vi "CREAT_SQL_TABLE.vi"() -> ()   [LabVIEW 2017]
uses:
  <vilib>/addons/database/Auxilliary.llb/DB Tools DataTypes.ctl
  <vilib>/addons/database/Connection.llb/DB Tools Open Connec (Path).vi
  <vilib>/addons/database/NI_Database_API.lvlib
panel:
  out "columns":string[](array[string])
  out "column information":T2(array[cluster])
  out "error out":errorcluster
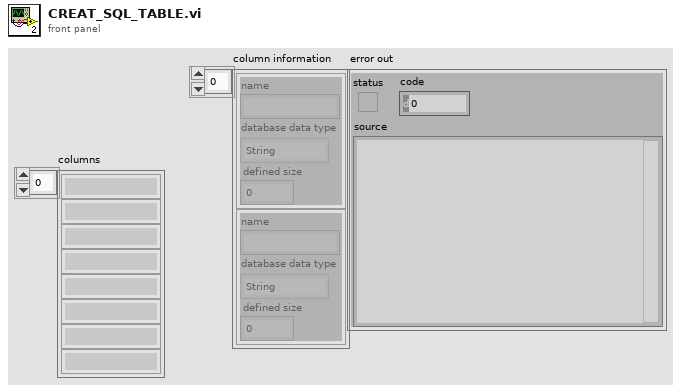
[diagram p1: front panel]
types:
  T1 = typedef "NI_Database_API.lvlib/DB Tools DataTypes.ctl" = enum16{"String", "Long (I32)", "Single (SGL)", "Double (DBL)", "Date/Time", "Binary"}
  T2 = cluster{"name":string, "database data type":T1, "defined size":i32}[]
  T3 = cluster{"name":string, "database data type":T1, "defined size":i32, "allow null?":bool}[]
  T4 = typedef "NI_Database_API.lvlib/Conn ObjectReference.ctl" = refnum<k1>
  T5 = cluster{"seconds since 1Jan1904":timestamp, "table":string, "table":string, "table":string}
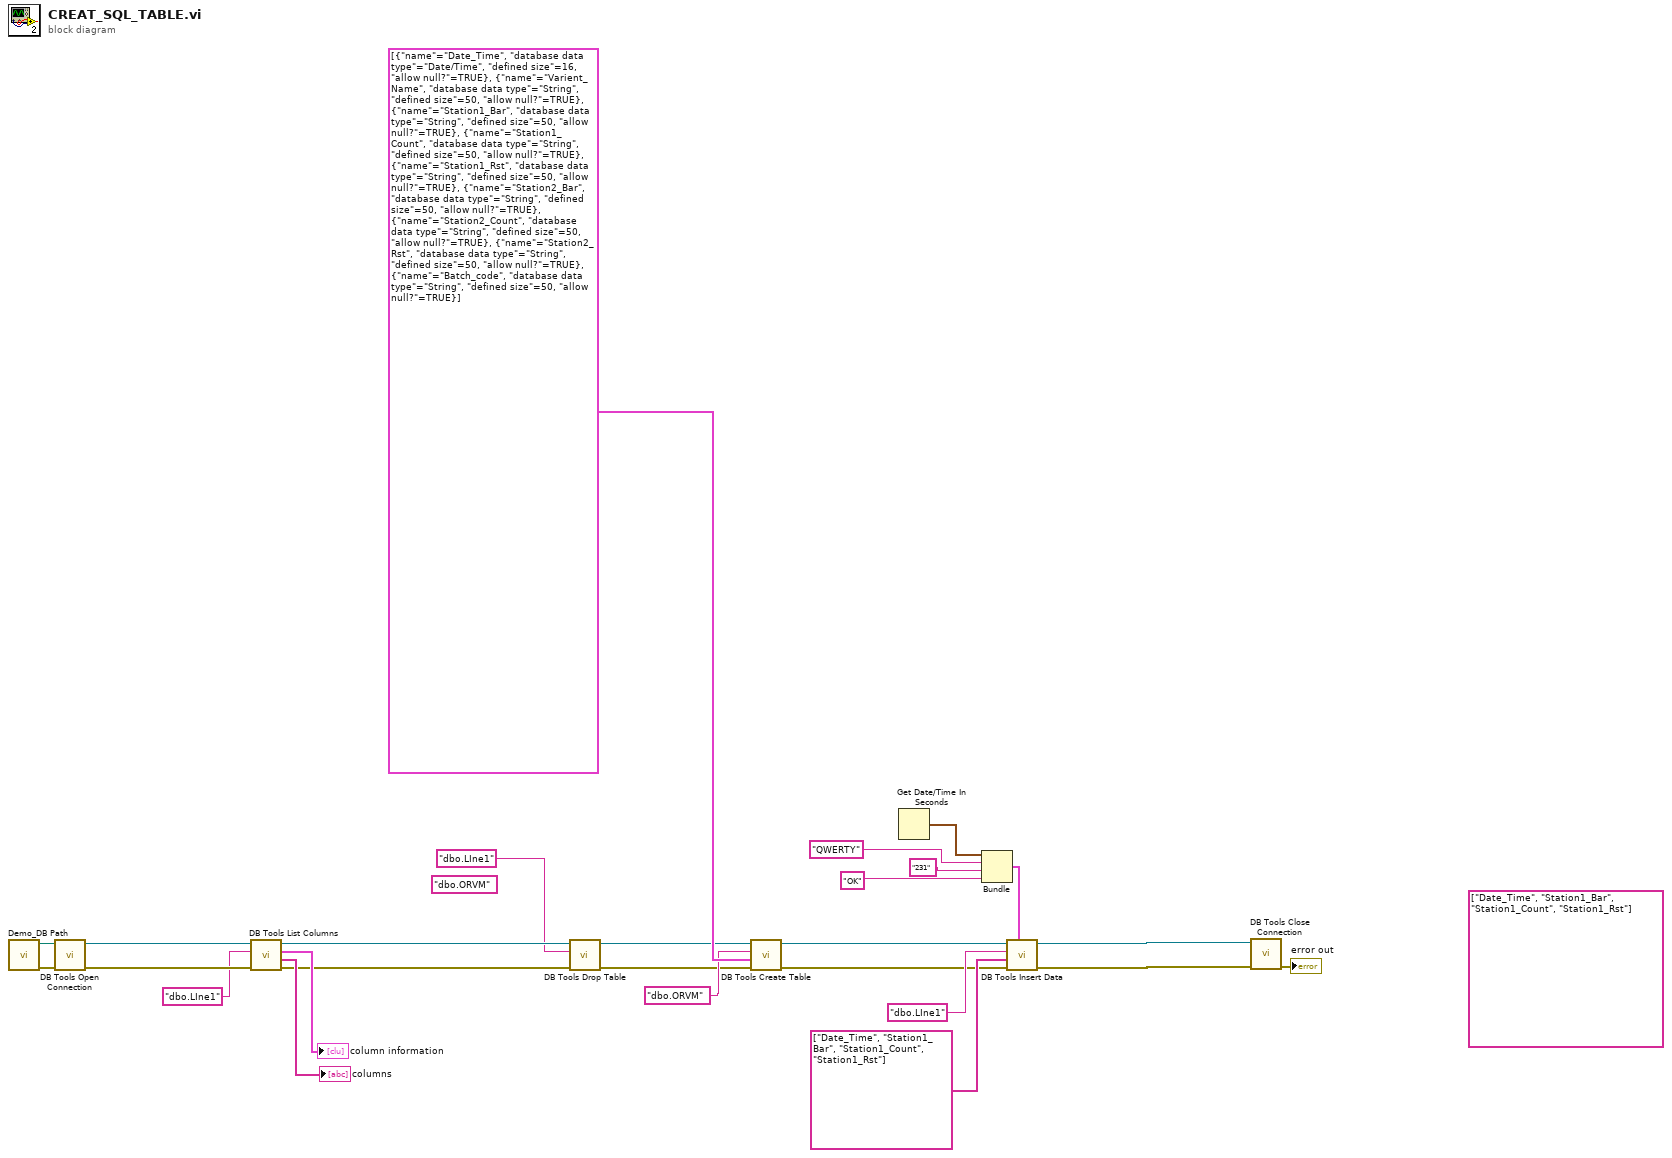
[diagram p0: block diagram]
diagram:
  (unwired) "dbo.ORVM" ("table")
  (unwired) string[] ["Date_Time", "Station1_Bar", "Station1_Count", "Station1_Rst"] ("columns")
  n1 = call "Demo_DB Path.vi"() -> ("error out"=w25:errorcluster, "DB Path"=w26:path)  [unwired: 10 in]
  n2 = call-poly <vilib>:"DB Tools Open Connection.vi"("error in (no error)"=w25, "connection information"=w26) -> ("error out"=w15:errorcluster, "connection reference"=w14:T4)  [unwired: 6 in]
  n3 = call <vilib>:"DB Tools List Columns.vi"("error in (no error)"=w15, "table"="dbo.LIne1", "connection reference"=w14) -> ("error out"=w3:errorcluster, "columns"=→"columns":string[], "column information"=→"column information":T2, "connection reference out"=w5:T4)  [unwired: 1 in]
  n4 = call <vilib>:"DB Tools Drop Table.vi"("error in (no error)"=w3, "table"="dbo.LIne1", "connection reference"=w5) -> ("error out"=w2:errorcluster, "connection reference out"=w4:T4)  [unwired: 5 in]
  n5 = call <vilib>:"DB Tools Create Table.vi"("error in (no error)"=w2, "column information"=T3 [{"name"="Date_Time", "database data type"=enum."Date/Time", "defined size"=16, "allow null?"=TRUE}, {"name"="Varient_Name", "database data type"=enum."String", "defined size"=50, "allow null?"=TRUE}, {"name"="Station1_Bar", "database data type"=enum."String", "defined size"=50, "allow null?"=TRUE}, {"name"="Station1_Count", "database data type"=enum."String", "defined size"=50, "allow null?"=TRUE}, {"name"="Station1_Rst", "database data type"=enum."String", "defined size"=50, "allow null?"=TRUE}, {"name"="Station2_Bar", "database data type"=enum."String", "defined size"=50, "allow null?"=TRUE}, {"name"="Station2_Count", "database data type"=enum."String", "defined size"=50, "allow null?"=TRUE}, {"name"="Station2_Rst", "database data type"=enum."String", "defined size"=50, "allow null?"=TRUE}, {"name"="Batch_code", "database data type"=enum."String", "defined size"=50, "allow null?"=TRUE}] ("output array"), "table"="dbo.ORVM", "connection reference"=w4) -> ("error out"=w10:errorcluster, "connection reference out"=w9:T4)  [unwired: 4 in]
  n6 = Get Date/Time In Seconds() -> (seconds since 1Jan1904=w20:timestamp)
  n7 = Bundle("seconds since 1Jan1904"=w20, "table"="QWERTY", "table"="231", "table"="OK") -> (w21:T5)  [unwired: 1 in]
  n8 = call <vilib>:"DB Tools Insert Data.vi"("data"=w21, "error in (no error)"=w10, "columns"=string[] ["Date_Time", "Station1_Bar", "Station1_Count", "Station1_Rst"] ("columns 2"), "table"="dbo.LIne1", "connection reference"=w9) -> ("error out"=w22:errorcluster, "connection reference out"=w23:T4)  [unwired: 5 in]
  n9 = call <vilib>:"DB Tools Close Connection.vi"("error in (no error)"=w22, "connection reference"=w23) -> ("error out"=→"error out":errorcluster)  [unwired: 5 in]
